vi "FIFO Flush.vi"(8 "Error In":errorcluster, 11 "FPGA VI Ref":T1) -> (0 "Error Out":errorcluster, 2 "Ch0 Elements Remaining":u32, 3 "FPGA VI Reference Out":T1)   [LabVIEW 2017]
uses:
  RIG-SPECIFIC FILES/FPGA Refs/FPGA Ref.ctl
  <vilib>/Utility/error.llb/Error Cluster From Error Code.vi
  <vilib>/rvi/errors/niLvFpgaAdjustHostInterfaceError.vi
  <vilib>/rvi/interface/nirviMethod/nirviMethod.xnode
  <vilib>/rvi/errors/niLvFpgaMergeErrorWithErrorCode.vi
  <vilib>/FPGAPlugInAG/Dynamic/niLvFpga_ReadFifo_Dynamic.vi
panel:
  out "Array":u32[](array[numeric])
  out "Image time zero":u32
  out "Data Image Time":u64[](array[numeric])
  out "Data Ch1":u32[](array[numeric])
  out "Ch1 Elements Remaining":u32
  out "Data Ch0":u32[](array[numeric])
  in  "Manual force stop":bool
  out "Loop":i32
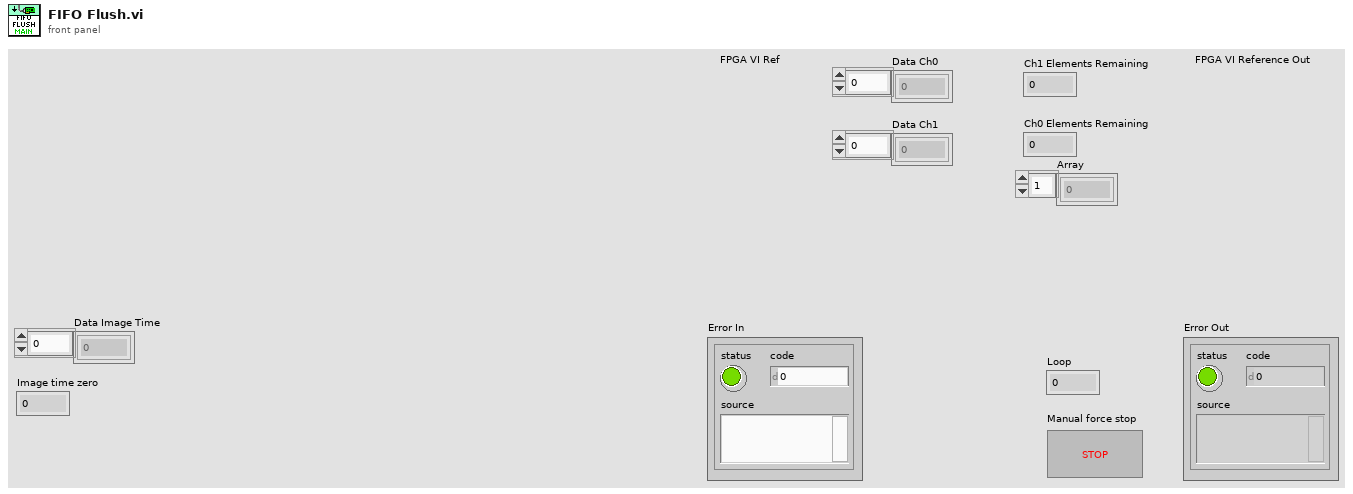
[diagram p1: front panel]
types:
  T1 = typedef "FPGA Ref.ctl" = refnum<k20>
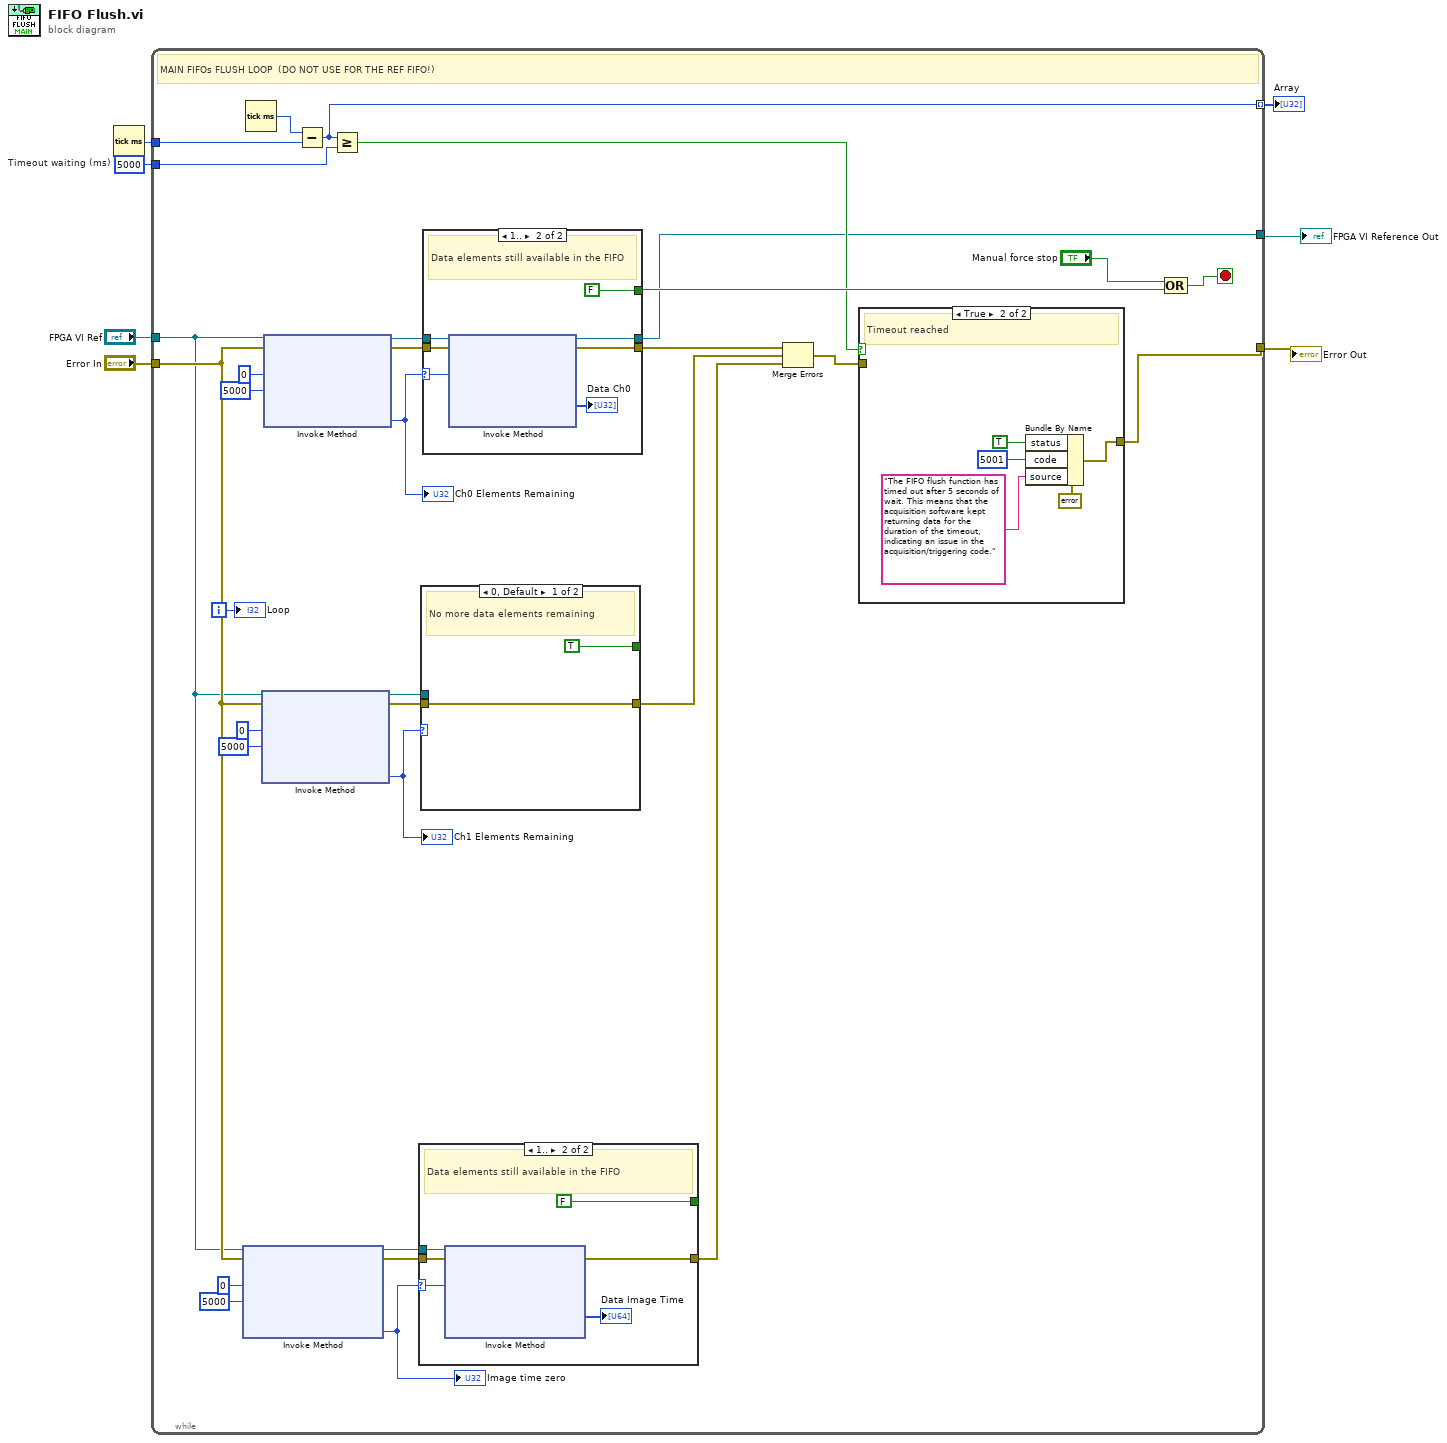
[diagram p0: block diagram]
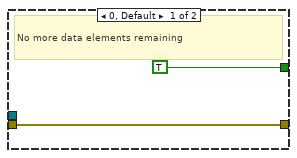
[diagram p2: hidden frame]
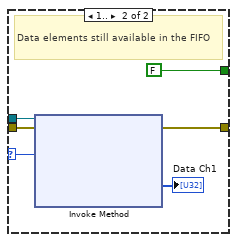
[diagram p3: hidden frame]
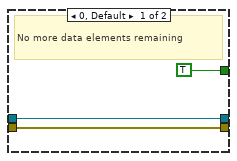
[diagram p5: hidden frame]
diagram:
  w5 = u32 5000  # Timeout waiting (ms)
  n1 = Tick Count (ms)() -> (millisecond timer value=w4:u32)
  n2 = while {
    tunnel: "Error In" -> [w10]
    tunnel: [w31] -> w6
    tunnel: w4 -> [w34]
    tunnel: w5 -> [w32]
    tunnel: "FPGA VI Ref" -> [w9]
    tunnel: [w17] -> w2
    tunnel: [w8] -> w1 mode=indexing
    i -> [w39]
    stop <- w38 stop-if-true
    # "MAIN FIFOs FLUSH LOOP  (DO NOT USE FOR THE REF FIFO!)"
    n3 = xnode "Invoke Method"("FPGA VI Reference In"=w9, "error in"=w10, "Number of Elements"=u32 0, "Timeout (ms)"=5000) -> ("FPGA VI Reference Out"=w15:T1, "error out"=w16:errorcluster, "Elements Remaining"=w12:u32)  [unwired: 1 out]
    "Image time zero" <- w12
    n4 = Tick Count (ms)() -> (millisecond timer value=w35:u32)
    n5 = xnode "Invoke Method"("FPGA VI Reference In"=w9, "error in"=w10, "Number of Elements"=u32 0, "Timeout (ms)"=5000) -> ("FPGA VI Reference Out"=w23:T1, "error out"=w22:errorcluster, "Elements Remaining"=w26:u32)  [unwired: 1 out]
    "Ch1 Elements Remaining" <- w26
    n6 = xnode "Invoke Method"("FPGA VI Reference In"=w9, "error in"=w10, "Number of Elements"=u32 0, "Timeout (ms)"=5000) -> ("FPGA VI Reference Out"=w36:T1, "error out"=w37:errorcluster, "Elements Remaining"=w27:u32)  [unwired: 1 out]
    "Ch0 Elements Remaining" <- w27
    n7 = Subtract(x=w35, y=w34) -> (x-y=w8:u32)
    n8 = Greater Or Equal?(x=w8, y=w32) -> (x >= y?=w18:bool)
    n9 = case shown="1.." w12 {
      selector: w12 -> [_ w44]
      tunnel: w16 -> [w40 w47]
      tunnel: w15 -> [_ w46]
      tunnel: [w40 w45] -> w11
      tunnel: [TRUE FALSE] -> _
      frame 0, Default {
        # "No more data elements remaining"
      }
      frame 1.. {
        # "Data elements still available in the FIFO"
        n10 = xnode "Invoke Method"("FPGA VI Reference In"=w46, "error in"=w47, "Number of Elements"=w44) -> ("error out"=w45:errorcluster, "Data"=→"Data Image Time":u64[])  [unwired: 1 in, 2 out]
      }
    }
    n11 = case shown="0, Default" w26 {
      selector: w26 -> [_ w52]
      tunnel: w22 -> [w48 w55]
      tunnel: w23 -> [_ w54]
      tunnel: [w48 w53] -> w21
      tunnel: [TRUE FALSE] -> _
      frame 0, Default {
        # "No more data elements remaining"
      }
      frame 1.. {
        # "Data elements still available in the FIFO"
        n12 = xnode "Invoke Method"("FPGA VI Reference In"=w54, "error in"=w55, "Number of Elements"=w52) -> ("error out"=w53:errorcluster, "Data"=→"Data Ch1":u32[])  [unwired: 1 in, 2 out]
      }
    }
    n13 = case shown="1.." w27 {
      selector: w27 -> [_ w68]
      tunnel: w37 -> [w63 w71]
      tunnel: w36 -> [w62 w70]
      tunnel: [w63 w69] -> w20
      tunnel: [TRUE FALSE] -> w33
      tunnel: [w62 w65] -> w17
      frame 0, Default {
        # "No more data elements remaining"
      }
      frame 1.. {
        # "Data elements still available in the FIFO"
        n14 = xnode "Invoke Method"("FPGA VI Reference In"=w70, "error in"=w71, "Number of Elements"=w68) -> ("FPGA VI Reference Out"=w65:T1, "error out"=w69:errorcluster, "Data"=→"Data Ch0":u32[])  [unwired: 1 in, 1 out]
      }
    }
    n15 = Merge Errors(w20, w21, w11) -> (w19:errorcluster)
    n16 = case shown="True" w18 {
      tunnel: w19 -> [w56 _]
      tunnel: [w56 w57] -> w31
      frame False {
      }
      frame True {
        # "Timeout reached"
        n17 = Bundle By Name(cluster=errorcluster {"status"=TRUE, "code"=5001, "source"=""} ("error out"), "status"=TRUE, "code"=5001, "source"="The FIFO flush function has timed out after 5 seconds of wait. This means that the acquisition software kept returning data for the duration of the timeout, indicating an issue in the acquisition/triggering code." ("Error Source")) -> (w57:errorcluster)
      }
    }
    n18 = Compound Arithmetic op=OR("Manual force stop", w33) -> (w38:bool)
    "Loop" <- w39
  }
  "Error Out" <- w6
  "FPGA VI Reference Out" <- w2
  "Array" <- w1
